vi "Error 5101 - Message Confirmation Not As Expected--const.vi"() -> (0 "error out":errorcluster)   [LabVIEW 2017, in "Communications Library.lvlib"]
doc: "Error 5101\n\nError sending a synchronous message to the DTACQ device. Expected to receive the terminating character (newline \\n) as a confirmation message, but a different message was received."
uses:
  Communications Library.lvlib
  <vilib>/Utility/error.llb/Error Cluster From Error Code.vi
  <vilib>/ErrorRing/Error Ring.xnode
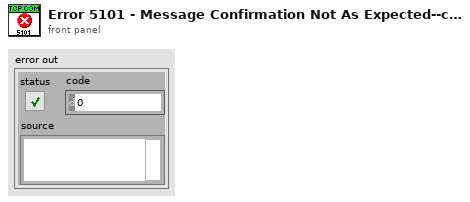
[diagram p1: front panel]
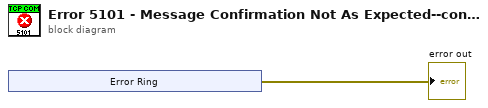
[diagram p0: block diagram]
diagram:
  n1 = xnode "Error Ring"() -> ("error out"=→"error out":errorcluster)
